vi "Run Debug Checklist.vi"(8 "error in (no error)":errorcluster, 11 "Data In":T2 {"Toggle Channels"."Initial State" items=["High"=101, "Low"=102]; "Sample Rate" format="%.2p"}) -> (0 "error out":errorcluster, 2 "Debugging Checklist":T1, 3 "Data Out":T2 {"Toggle Channels"."Initial State" items=["High"=101, "Low"=102]; "Sample Rate" format="%.2p"})   [LabVIEW 2024]
uses:
  Controls/Debugging Checklist.ctl
  Controls/Script Trigger Routing.ctl
  Controls/Toggle Channel.ctl
  Controls/Data.ctl
  <vilib>/regexp/Match Regular Expression.xnode
  72063e7b-09d2-4d39-9c85-2e0e457aba84.vi
  951ec342-c686-4d31-a251-473d83e5815b.vi
  d486b57b-f3ef-4cf1-a696-9a60b6fd83b1.vi
  c6059185-f7f4-417c-bbd4-247f5af7741b.vi
  03b6714b-2279-4eb4-9697-7dd13d22bb94.vi
  244f46ae-2737-4380-a61e-589f98d331e5.vi
  3385c125-95ec-4038-930b-a55a0d2c3c58.vi
  9be64401-7d23-4708-ad72-c1a8af7e7189.vi
  50adc59f-fe99-4d35-9e3d-f38453d61c5f.vi
panel:
  out "Used Names":set{string}(c389)
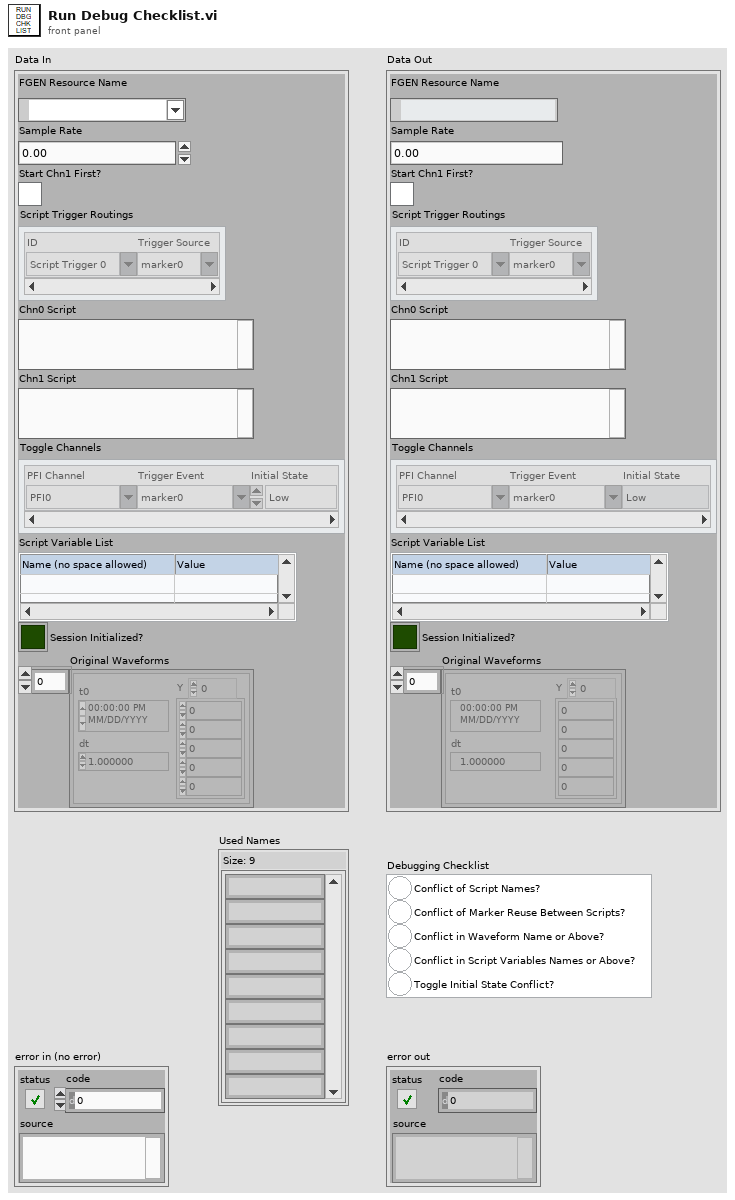
[diagram p1: front panel]
types:
  T1 = typedef "Debugging Checklist.ctl" = cluster{"Conflict of Script Names?":bool, "Conflict of Marker Reuse Between Scripts?":bool, "Conflict in Waveform Name or Above?":bool, "Conflict in Script Variables Names or Above?":bool, "Toggle Initial State Conflict?":bool}
  T2 = typedef "Data.ctl" = cluster{"FGEN Resource Name":refnum<k15>, "Sample Rate":dbl, "Start Chn1 First?":bool, "Script Trigger Routings":T3[], "Chn0 Script":string, "Chn1 Script":string, "Toggle Channels":T4[], "Script Variable List":string[][], "Session Initialized?":bool, "Original Waveforms":waveform(dbl)[]}
  T3 = typedef "Script Trigger Routing.ctl" = cluster{"ID":string, "Trigger Source":string}
  T4 = typedef "Toggle Channel.ctl" = cluster{"PFI Channel":string, "Trigger Event":string, "Initial State":u16}
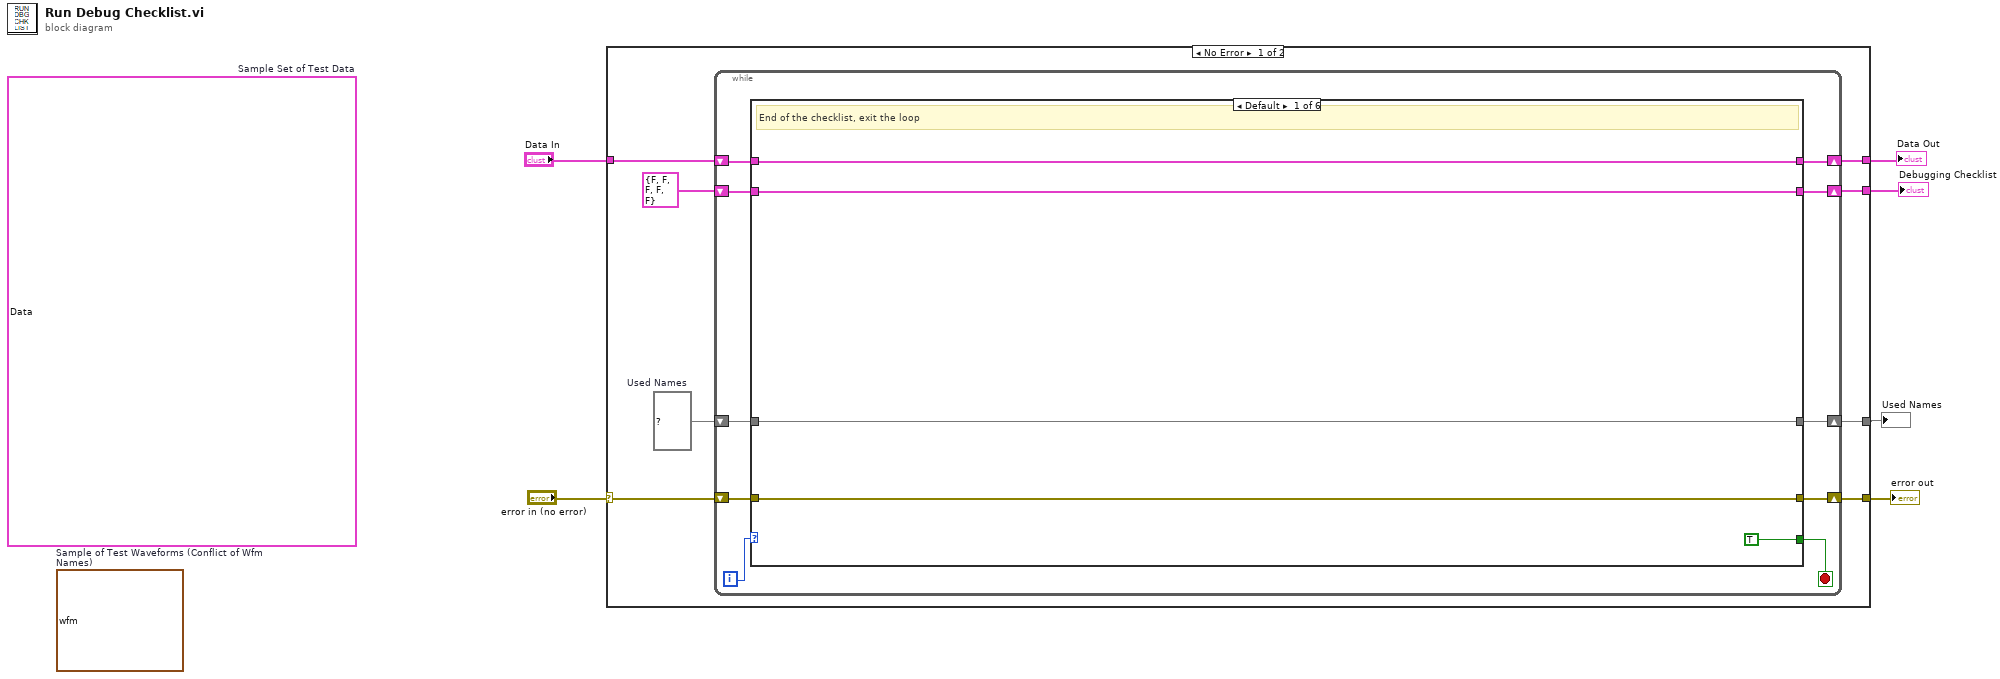
[diagram p0: block diagram]
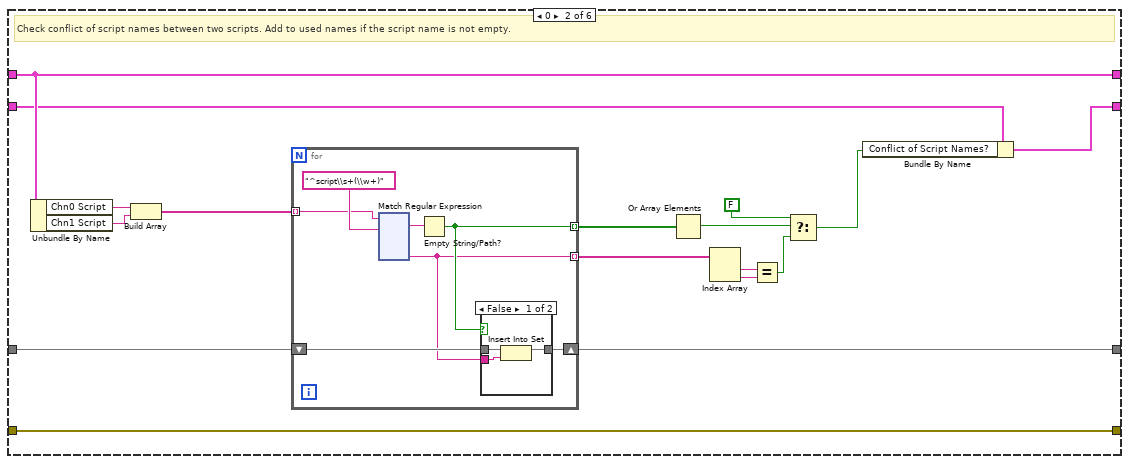
[diagram p2: hidden frame]
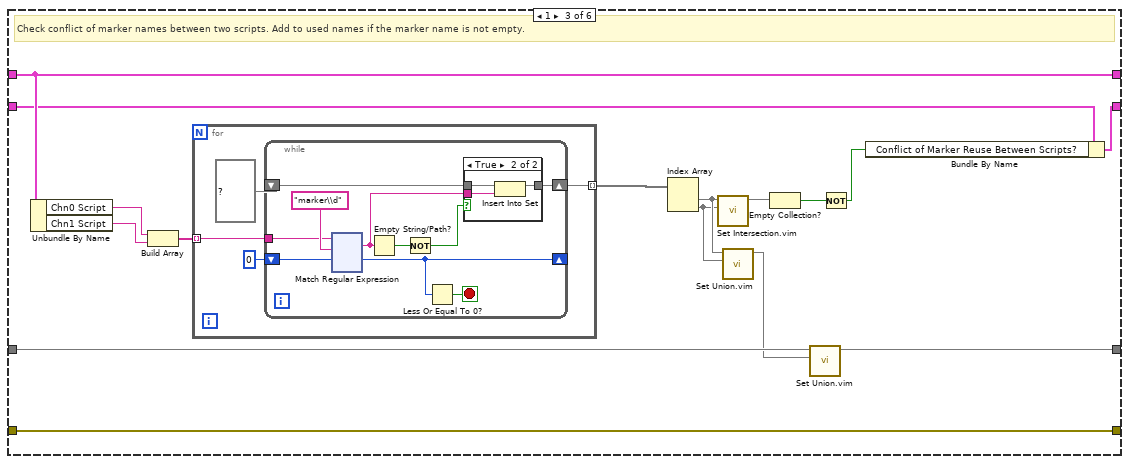
[diagram p4: hidden frame]
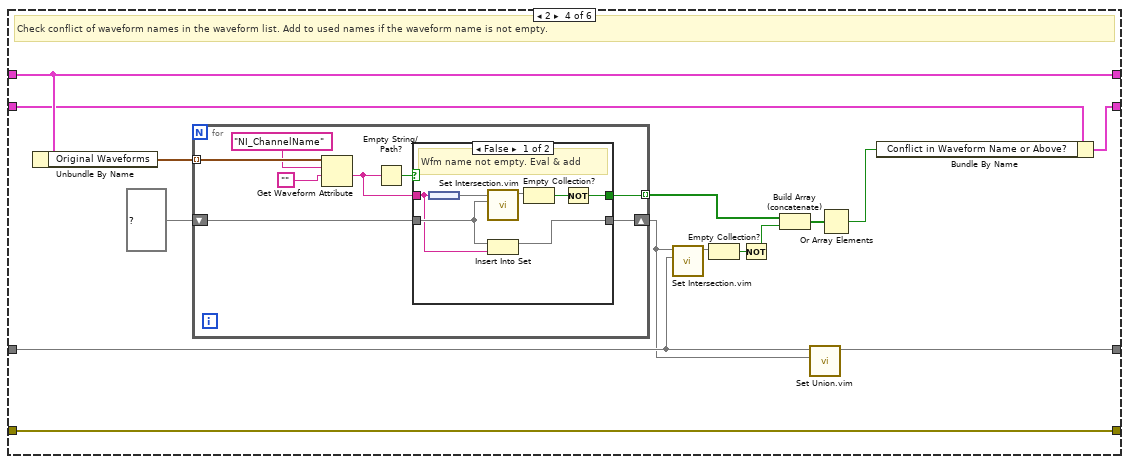
[diagram p6: hidden frame]
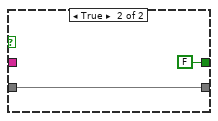
[diagram p7: hidden frame]
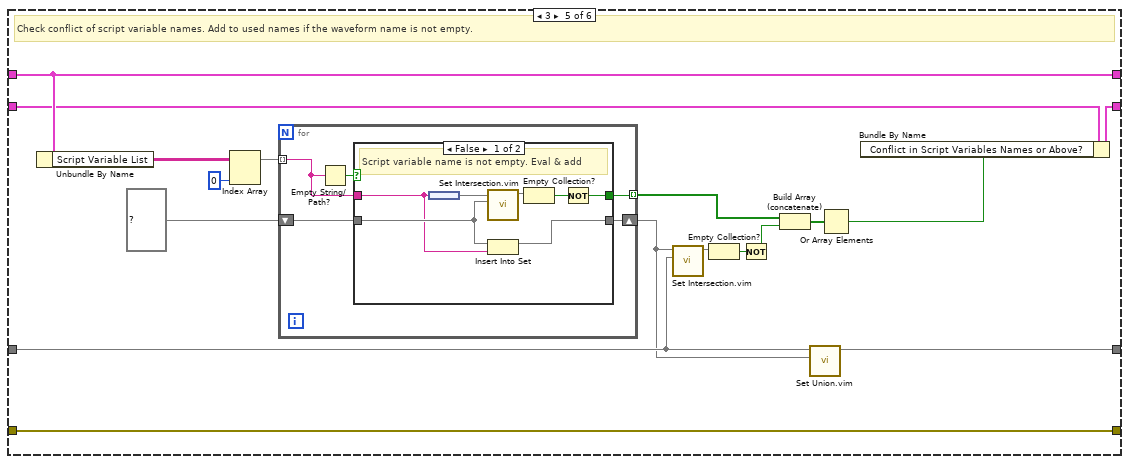
[diagram p8: hidden frame]
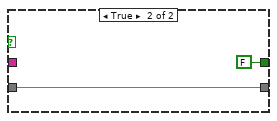
[diagram p9: hidden frame]
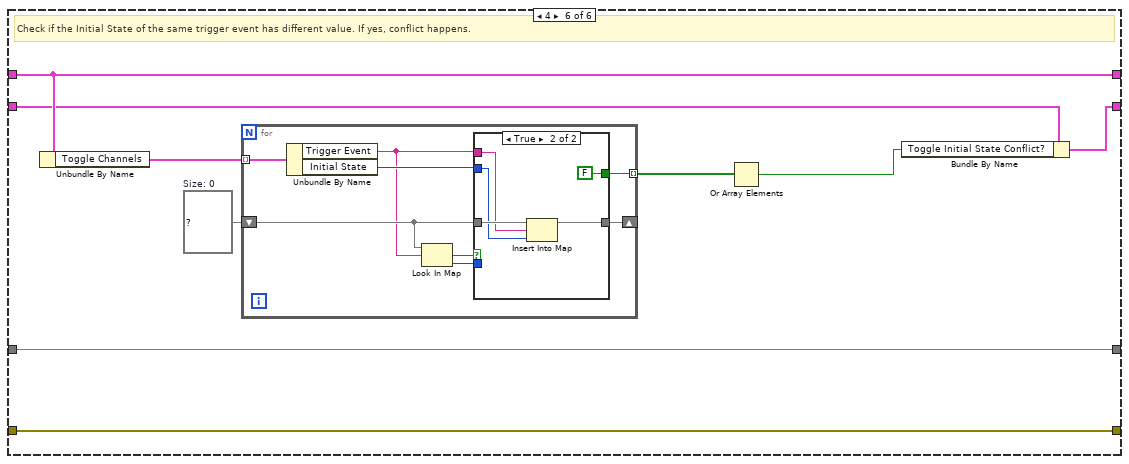
[diagram p10: hidden frame]
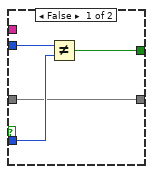
[diagram p11: hidden frame]
diagram:
  (unwired) waveform(dbl)[] [{"t0"=timestamp(0 s since 1904-01-01), "dt"=1e-06, "Y"=[0.0, 0.0, 0.0, 0.0, 0.0, 0.0, 0.0, 0.0, 0.0, 0.0], "attributes"=variant("NI_ChannelName"=variant(string "DcOff10us"), "NI_ExpIsRelativeTime"=variant(bool TRUE), "NI_ExpStartTimeStamp"=variant(timestamp timestamp(3848540379.749288 s since 1904-01-01)), "NI_ExpTimeStamp"=variant(timestamp timestamp(3848540379.749288 s since 1904-01-01)), "NI_ExpXDimension"=variant(string "t"))}, {"t0"=timestamp(0 s since 1904-01-01), "dt"=1e-06, "Y"=[3.3, 3.3, 3.3, 3.3, 3.3, 3.3, 3.3, 3.3, 3.3, 3.3, 3.3, 3.3, 3.3, 3.3, 3.3, 3.3, 3.3, 3.3, 3.3, 3.3, 3.3, 3.3, 3.3, 3.3, 3.3, 3.3, 3.3, 3.3, 3.3, 3.3, 3.3, 3.3, 3.3, 3.3, 3.3, 3.3, 3.3, 3.3, 3.3, 3.3, 3.3, 3.3, 3.3, 3.3, 3.3, 3.3, 3.3, 3.3, 3.3, 3.3, 3.3, 3.3, 3.3, 3.3, 3.3, 3.3, 3.3, 3.3, 3.3, 3.3, 3.3, 3.3, 3.3, 3.3, 3.3, 3.3, 3.3, 3.3, 3.3, 3.3, 3.3, 3.3, 3.3, 3.3, 3.3, 3.3, 3.3, 3.3, 3.3, 3.3, 3.3, 3.3, 3.3, 3.3, 3.3, 3.3, 3.3, 3.3, 3.3, 3.3, 3.3, 3.3, 3.3, 3.3, 3.3, 3.3, 3.3, 3.3, 3.3, 3.3, 3.3, 3.3, 3.3, 3.3, 3.3, 3.3, 3.3, 3.3, 3.3, 3.3, 3.3, 3.3, 3.3, 3.3, 3.3, 3.3, 3.3, 3.3, 3.3, 3.3], "attributes"=variant("NI_ChannelName"=variant(string "DcOn120us"), "NI_ExpIsRelativeTime"=variant(bool TRUE), "NI_ExpStartTimeStamp"=variant(timestamp timestamp(3848540379.749288 s since 1904-01-01)), "NI_ExpTimeStamp"=variant(timestamp timestamp(3848540379.749288 s since 1904-01-01)), "NI_ExpXDimension"=variant(string "t"))}, {"t0"=timestamp(0 s since 1904-01-01), "dt"=5e-08, "Y"=array[2000 elements], "attributes"=variant("NI_ChannelName"=variant(string "DcOff10us"), "NI_ExpIsRelativeTime"=variant(bool TRUE), "NI_ExpStartTimeStamp"=variant(timestamp timestamp(3848540379.7482686 s since 1904-01-01)), "NI_ExpTimeStamp"=variant(timestamp timestamp(3848540379.7482686 s since 1904-01-01)), "NI_ExpXDimension"=variant(string "t"))}]  # Sample of Test Waveforms (Conflict of Wfm Names)
  (unwired) T2 {"FGEN Resource Name"="", "Sample Rate"=20000000.0, "Start Chn1 First?"=FALSE, "Script Trigger Routings"=[], "Chn0 Script"="script myScript1\n  Generate DcOff10us\n  Generate DcOn120us marker0(tON1, tOFF1) marker1(tON2, tOFF2)\n  Generate DcOff10us\nend script", "Chn1 Script"="script myScript2\n  Wait until scriptTrigger0\n  Generate Sine1kHz100us\n  Generate DcOff10us\nend script", "Toggle Channels"=[], "Script Variable List"=[["ABC", "1"], ["myScript2", "2"], ["DcOff10us", "3"]], "Session Initialized?"=FALSE, "Original Waveforms"=[{"t0"=timestamp(0 s since 1904-01-01), "dt"=1e-06, "Y"=[0.0, 0.0, 0.0, 0.0, 0.0, 0.0, 0.0, 0.0, 0.0, 0.0], "attributes"=variant("NI_ChannelName"=variant(string "DcOff10us"), "NI_ExpIsRelativeTime"=variant(bool TRUE), "NI_ExpStartTimeStamp"=variant(timestamp timestamp(3848034048.1076193 s since 1904-01-01)), "NI_ExpTimeStamp"=variant(timestamp timestamp(3848034048.1076193 s since 1904-01-01)), "NI_ExpXDimension"=variant(string "t"))}, {"t0"=timestamp(0 s since 1904-01-01), "dt"=1e-06, "Y"=[3.3, 3.3, 3.3, 3.3, 3.3, 3.3, 3.3, 3.3, 3.3, 3.3, 3.3, 3.3, 3.3, 3.3, 3.3, 3.3, 3.3, 3.3, 3.3, 3.3, 3.3, 3.3, 3.3, 3.3, 3.3, 3.3, 3.3, 3.3, 3.3, 3.3, 3.3, 3.3, 3.3, 3.3, 3.3, 3.3, 3.3, 3.3, 3.3, 3.3, 3.3, 3.3, 3.3, 3.3, 3.3, 3.3, 3.3, 3.3, 3.3, 3.3, 3.3, 3.3, 3.3, 3.3, 3.3, 3.3, 3.3, 3.3, 3.3, 3.3, 3.3, 3.3, 3.3, 3.3, 3.3, 3.3, 3.3, 3.3, 3.3, 3.3, 3.3, 3.3, 3.3, 3.3, 3.3, 3.3, 3.3, 3.3, 3.3, 3.3, 3.3, 3.3, 3.3, 3.3, 3.3, 3.3, 3.3, 3.3, 3.3, 3.3, 3.3, 3.3, 3.3, 3.3, 3.3, 3.3, 3.3, 3.3, 3.3, 3.3, 3.3, 3.3, 3.3, 3.3, 3.3, 3.3, 3.3, 3.3, 3.3, 3.3, 3.3, 3.3, 3.3, 3.3, 3.3, 3.3, 3.3, 3.3, 3.3, 3.3], "attributes"=variant("NI_ChannelName"=variant(string "DcOn120us"), "NI_ExpIsRelativeTime"=variant(bool TRUE), "NI_ExpStartTimeStamp"=variant(timestamp timestamp(3848034048.1076193 s since 1904-01-01)), "NI_ExpTimeStamp"=variant(timestamp timestamp(3848034048.1076193 s since 1904-01-01)), "NI_ExpXDimension"=variant(string "t"))}, {"t0"=timestamp(0 s since 1904-01-01), "dt"=5e-08, "Y"=array[2000 elements], "attributes"=variant("NI_ChannelName"=variant(string "Sine1kHz100us"), "NI_ExpIsRelativeTime"=variant(bool TRUE), "NI_ExpStartTimeStamp"=variant(timestamp timestamp(3848034048.1066246 s since 1904-01-01)), "NI_ExpTimeStamp"=variant(timestamp timestamp(3848034048.1066246 s since 1904-01-01)), "NI_ExpXDimension"=variant(string "t"))}]}  # Sample Set of Test Data
  n1 = case shown="No Error" "error in (no error)" {
    selector: "error in (no error)" -> [w11 w418]
    tunnel: "Data In" -> [w13 w417]
    tunnel: [w12 w417] -> w5
    tunnel: [w10 w418] -> w3
    tunnel: [w14 _] -> w2
    tunnel: [w8 _] -> w1
    frame No Error {
      w7 = set{string} {}  # Used Names
      n2 = while {
        shift-right: [w22] -> w12
        shift-left: w13 -> [w23]
        shift-right: [w20] -> w10
        shift-left: w11 -> [w21]
        shift-right: [w24] -> w14
        shift-left: T1 {"Conflict of Script Names?"=FALSE, "Conflict of Marker Reuse Between Scripts?"=FALSE, "Conflict in Waveform Name or Above?"=FALSE, "Conflict in Script Variables Names or Above?"=FALSE, "Toggle Initial State Conflict?"=FALSE} ("Debugging") -> [w18]
        shift-right: [w15] -> w8
        shift-left: w7 -> [w17]
        i -> [w19]
        stop <- w16 stop-if-true
        n3 = case shown="Default" w19 {
          tunnel: [w27 w46 w192 w342 w376 w399] -> w24
          tunnel: w23 -> [w29 w44 w191 w341 w375 w398]
          tunnel: [w29 w44 w191 w341 w375 w398] -> w22
          tunnel: w21 -> [w28 w43 w190 w340 w374 w397]
          tunnel: [w28 w43 w190 w340 w374 w397] -> w20
          tunnel: w18 -> [w27 w42 w189 w339 w373 w396]
          tunnel: w17 -> [w25 w31 w179 w331 w365 w394]
          tunnel: [TRUE _ _ _ _ _] -> w16
          tunnel: [w25 w30 w177 w337 w371 w394] -> w15
          frame Default {
            # "End of the checklist, exit the loop"
          }
          frame 0 {
            # "Check conflict of script names between two scripts. Add to used names if the script name is not empty."
            n4 = Unbundle By Name(w44) -> ("Chn0 Script"=w45:string, "Chn1 Script"=w37:string)
            n5 = Build Array(w45, w37) -> (w38:string[])
            n6 = for {
              tunnel: [w49] -> w39 mode=indexing
              tunnel: [w47] -> w35 mode=indexing
              tunnel: w38 -> [w51] mode=indexing
              shift-right: [w48] -> w30
              shift-left: w31 -> [w50]
              n7 = xnode "Match Regular Expression"("input string"=w51, "regular expression"="^script\\s+(\\w+)") -> ("whole match"=w52:string, "submatch 1"=w47:string)  [unwired: 4 in, 4 out]
              n8 = Empty String/Path?(string/path=w52) -> (empty?=w49:bool)
              n9 = case shown="False" w49 {
                tunnel: w50 -> [w56 w57]
                tunnel: [w55 w57] -> w48
                tunnel: w47 -> [w54 _]
                frame False {
                  n10 = Insert Into Set(10:w54, 11:w56) -> (3:w55:set{string})  [unwired: 1 out]
                }
                frame True {
                }
              }
            }
            n11 = Or Array Elements(Boolean array=w39) -> (logical OR=w36:bool)
            n12 = Index Array(array=w35) -> (element #1=w34:string, element #2=w33:string)  [unwired: 2 in]
            n13 = Equal?(x=w34, y=w33) -> (x = y?=w32:bool)
            n14 = Select(t=FALSE, s=w36, f=w32) -> (s? t:f=w41:bool)
            n15 = Bundle By Name(cluster=w42, "Conflict of Script Names?"=w41) -> (w46:T1)
          }
          frame 1 {
            # "Check conflict of marker names between two scripts. Add to used names if the marker name is not empty."
            n16 = Unbundle By Name(w191) -> ("Chn0 Script"=w188:string, "Chn1 Script"=w186:string)
            n17 = Build Array(w188, w186) -> (w187:string[])
            n18 = for {
              tunnel: w187 -> [w195] mode=indexing
              tunnel: [w193] -> w185 mode=indexing
              n19 = while {
                tunnel: w195 -> [w205]
                shift-right: [w202] -> _
                shift-left: 0 ("offset past match") -> [w204]
                shift-right: [w200] -> w193
                shift-left: set{string} {} ("set in") -> [w199]
                stop <- w203 stop-if-true
                n20 = xnode "Match Regular Expression"("input string"=w205, "regular expression"="marker\\d", "offset (0)"=w204) -> ("whole match"=w197:string, "offset past match"=w202:i32)  [unwired: 3 in, 3 out]
                n21 = Empty String/Path?(string/path=w197) -> (empty?=w201:bool)
                n22 = Not(x=w201) -> (.not. x?=w198:bool)
                n23 = Less Or Equal To 0?(x=w202) -> (x <= 0?=w203:bool)
                n24 = case shown="True" w198 {
                  tunnel: [w207 w210] -> w200
                  tunnel: w199 -> [w207 w209]
                  tunnel: w197 -> [_ w208]
                  frame False {
                  }
                  frame True {
                    n25 = Insert Into Set(10:w208, 11:w209) -> (3:w210:set{string})  [unwired: 1 out]
                  }
                }
              }
            }
            n26 = Index Array(array=w185) -> (element #1=w181:set{string}, element #2=w180:set{string})  [unwired: 2 in]
            n27 = call "Set Intersection.vim"("set 2"=w180, "set 1"=w181) -> ("intersection"=w184:set{string})  [unwired: 9 in]
            n28 = call "Set Union.vim"("set 2"=w180, "set 1"=w181) -> ("union"=w178:set{string})  [unwired: 9 in]
            n29 = Empty Collection?(1:w184) -> (0:w183:bool)
            n30 = call "Set Union.vim"("set 2"=w178, "set 1"=w179) -> ("union"=w177:set{string})  [unwired: 9 in]
            n31 = Not(x=w183) -> (.not. x?=w182:bool)
            n32 = Bundle By Name(cluster=w189, "Conflict of Marker Reuse Between Scripts?"=w182) -> (w192:T1)
          }
          frame 2 {
            # "Check conflict of waveform names in the waveform list. Add to used names if the waveform name is not empty."
            n33 = Unbundle By Name(w341) -> ("Original Waveforms"=w336:waveform(dbl)[])
            n34 = for {
              tunnel: w336 -> [w350] mode=indexing
              shift-right: [w344] -> w328
              shift-left: set{string} {} ("Used Names") -> [w346]
              tunnel: [w343] -> w334 mode=indexing
              n35 = Get Waveform Attribute(5:"", 6:"NI_ChannelName" ("name"), 7:w350) -> (1:w345:string)  [unwired: 1 in, 3 out]
              n36 = Empty String/Path?(string/path=w345) -> (empty?=w347:bool)
              n37 = case shown="False" w347 {
                tunnel: w346 -> [w355 w358]
                tunnel: w345 -> [w354 _]
                tunnel: [w353 w358] -> w344
                tunnel: [w351 FALSE] -> w343
                frame False {
                  # "Wfm name not empty. Eval & add"
                  n38 = node(w354) -> (w356:set{string})
                  n39 = call "Set Intersection.vim"("set 2"=w355, "set 1"=w356) -> ("intersection"=w357:set{string})  [unwired: 9 in]
                  n40 = Insert Into Set(10:w354, 11:w355) -> (3:w353:set{string})  [unwired: 1 out]
                  n41 = Empty Collection?(1:w357) -> (0:w352:bool)
                  n42 = Not(x=w352) -> (.not. x?=w351:bool)
                }
                frame True {
                }
              }
            }
            n43 = call "Set Intersection.vim"("set 2"=w331, "set 1"=w328) -> ("intersection"=w332:set{string})  [unwired: 9 in]
            n44 = Empty Collection?(1:w332) -> (0:w333:bool)
            n45 = Not(x=w333) -> (.not. x?=w329:bool)
            n46 = Build Array (concatenate)(w334, w329) -> (w330:bool[])
            n47 = call "Set Union.vim"("set 2"=w328, "set 1"=w331) -> ("union"=w337:set{string})  [unwired: 9 in]
            n48 = Or Array Elements(Boolean array=w330) -> (logical OR=w338:bool)
            n49 = Bundle By Name(cluster=w339, "Conflict in Waveform Name or Above?"=w338) -> (w342:T1)
          }
          frame 3 {
            # "Check conflict of script variable names. Add to used names if the waveform name is not empty."
            n50 = Unbundle By Name(w375) -> ("Script Variable List"=w370:string[][])
            n51 = Index Array(array=w370, index (col)=0 ("disabled index (col)")) -> (element=w361:string[])  [unwired: 1 in]
            n52 = for {
              tunnel: w361 -> [w381] mode=indexing
              shift-right: [w378] -> w362
              shift-left: set{string} {} ("Used Names") -> [w379]
              tunnel: [w377] -> w368 mode=indexing
              n53 = Empty String/Path?(string/path=w381) -> (empty?=w380:bool)
              n54 = case shown="False" w380 {
                tunnel: w379 -> [w386 w389]
                tunnel: w381 -> [w385 _]
                tunnel: [w384 w389] -> w378
                tunnel: [w382 FALSE] -> w377
                frame False {
                  # "Script variable name is not empty. Eval & add"
                  n55 = node(w385) -> (w387:set{string})
                  n56 = call "Set Intersection.vim"("set 2"=w386, "set 1"=w387) -> ("intersection"=w388:set{string})  [unwired: 9 in]
                  n57 = Insert Into Set(10:w385, 11:w386) -> (3:w384:set{string})  [unwired: 1 out]
                  n58 = Empty Collection?(1:w388) -> (0:w383:bool)
                  n59 = Not(x=w383) -> (.not. x?=w382:bool)
                }
                frame True {
                }
              }
            }
            n60 = call "Set Intersection.vim"("set 2"=w365, "set 1"=w362) -> ("intersection"=w366:set{string})  [unwired: 9 in]
            n61 = Empty Collection?(1:w366) -> (0:w367:bool)
            n62 = Not(x=w367) -> (.not. x?=w363:bool)
            n63 = Build Array (concatenate)(w368, w363) -> (w364:bool[])
            n64 = call "Set Union.vim"("set 2"=w362, "set 1"=w365) -> ("union"=w371:set{string})  [unwired: 9 in]
            n65 = Or Array Elements(Boolean array=w364) -> (logical OR=w372:bool)
            n66 = Bundle By Name(cluster=w373, "Conflict in Script Variables Names or Above?"=w372) -> (w376:T1)
          }
          frame 4 {
            w392 = map{string, u16} {}  # Size: 0
            # "Check if the Initial State of the same trigger event has different value. If yes, conflict happens."
            n67 = Unbundle By Name(w398) -> ("Toggle Channels"=w393:T4[])
            n68 = for {
              tunnel: w393 -> [w407] mode=indexing
              shift-right: [w405] -> _
              shift-left: w392 -> [w404]
              tunnel: [w400] -> w391 mode=indexing
              n69 = Unbundle By Name(w407) -> ("Trigger Event"=w403:string, "Initial State"=w406:u16)
              n70 = Look In Map(map=w404, key=w403) -> (key not found?=w402:bool, value=w401:u16)  [unwired: 1 in]
              n71 = case shown="True" w402 {
                tunnel: w406 -> [w411 w413]
                tunnel: [w408 w416] -> w405
                tunnel: w404 -> [w408 w415]
                tunnel: w403 -> [_ w414]
                tunnel: w401 -> [w410 _]
                tunnel: [w409 FALSE] -> w400
                frame False {
                  n72 = Not Equal?(x=w411, y=w410) -> (x != y?=w409:bool)
                }
                frame True {
                  n73 = Insert Into Map(map in=w415, key=w414, value=w413) -> (map out=w416:map{string, u16})  [unwired: 2 out]
                }
              }
            }
            n74 = Or Array Elements(Boolean array=w391) -> (logical OR=w395:bool)
            n75 = Bundle By Name(cluster=w396, "Toggle Initial State Conflict?"=w395) -> (w399:T1)
          }
        }
      }
    }
    frame Error {
    }
  }
  "Data Out" <- w5
  "error out" <- w3
  "Debugging Checklist" <- w2
  "Used Names" <- w1
